vi "Configure Trigger.vi"   [LabVIEW 2009, in "Tektronix DPO MSO 2000 4000 Series.lvlib"]
doc: "Select a trigger type for an oscilloscope and configures trigger type settings. The available trigger types includes:\nEdge Trigger\nPulse Width Trigger\nRunt Trigger\nLogic Trigger\nSetup & Hold Trigger\nRise Fall Time Trigger\nVideo Trigger\nI2C Trigger\nSPI Trigger\nCAN Trigger\nProbe Trigger"
uses:
  <instrlib>/Tektronix DPO MSO 2000 4000 Series/Tektronix DPO MSO 2000 4000 Series.lvlib
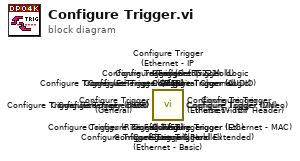
[diagram p0: block diagram]
diagram:
  n1 = call <instrlib>:"Configure Trigger (External).vi"() -> ()  [unwired: 14 in, 2 out]
  n2 = call <instrlib>:"Configure Trigger (Logic & Digital Channel).vi"() -> ()  [unwired: 14 in, 2 out]
  n3 = call <instrlib>:"Configure Trigger (General).vi"() -> ()  [unwired: 14 in, 2 out]
  n4 = call <instrlib>:"Configure Trigger (Ethernet - TCP Header).vi"() -> ()  [unwired: 14 in, 2 out]
  n5 = call <instrlib>:"Configure Trigger (Ethernet - QTAG).vi"() -> ()  [unwired: 14 in, 2 out]
  n6 = call <instrlib>:"Configure Trigger (Ethernet - MAC).vi"() -> ()  [unwired: 14 in, 2 out]
  n7 = call <instrlib>:"Configure Trigger (Ethernet - IP Header).vi"() -> ()  [unwired: 14 in, 2 out]
  n8 = call <instrlib>:"Configure Trigger (Ethernet - Data).vi"() -> ()  [unwired: 14 in, 2 out]
  n9 = call <instrlib>:"Configure Trigger (Ethernet - Basic).vi"() -> ()  [unwired: 14 in, 2 out]
  n10 = call <instrlib>:"Configure Trigger (USB).vi"() -> ()  [unwired: 14 in, 2 out]
  n11 = call <instrlib>:"Configure Trigger (LIN).vi"() -> ()  [unwired: 14 in, 2 out]
  n12 = call <instrlib>:"Configure Trigger (AUDIO).vi"() -> ()  [unwired: 14 in, 2 out]
  n13 = call <instrlib>:"Configure Trigger (Parallel).vi"() -> ()  [unwired: 14 in, 2 out]
  n14 = call <instrlib>:"Configure Trigger (RS232).vi"() -> ()  [unwired: 14 in, 2 out]
  n15 = call <instrlib>:"Configure Trigger (CAN).vi"() -> ()  [unwired: 14 in, 2 out]
  n16 = call <instrlib>:"Configure Trigger (SPI).vi"() -> ()  [unwired: 14 in, 2 out]
  n17 = call <instrlib>:"Configure Trigger (I2C).vi"() -> ()  [unwired: 14 in, 2 out]
  n18 = call <instrlib>:"Configure Trigger (Video).vi"() -> ()  [unwired: 14 in, 2 out]
  n19 = call <instrlib>:"Configure Trigger (Rise Fall Time).vi"() -> ()  [unwired: 14 in, 2 out]
  n20 = call <instrlib>:"Configure Trigger (Setup & Hold Extended).vi"() -> ()  [unwired: 14 in, 2 out]
  n21 = call <instrlib>:"Configure Trigger (Setup & Hold).vi"() -> ()  [unwired: 14 in, 2 out]
  n22 = call <instrlib>:"Configure Trigger (Logic).vi"() -> ()  [unwired: 14 in, 2 out]
  n23 = call <instrlib>:"Configure Trigger (Runt).vi"() -> ()  [unwired: 14 in, 2 out]
  n24 = call <instrlib>:"Configure Trigger (Pulse Width).vi"() -> ()  [unwired: 14 in, 2 out]
  n25 = call <instrlib>:"Configure Trigger (Edge).vi"() -> ()  [unwired: 14 in, 2 out]
